vi "FUG_MagnetPS.destructor.vi"(0 "i ref in":refnum<vi>, 5 "error in (no error)":errorcluster) -> (19 "error out":errorcluster)   [LabVIEW 2014, in "FUG_MagnetPS.lvlib"]
doc: "This is the destructor of a class.\n\nLicense Agreement for this software:\n\nCopyright (C)\nGesellschaft für Schwerionenforschung, GSI\nPlanckstr. 1\n64291 Darmstadt\nGermany\n\nContact: D.Beck@gsi.de \n\nThis program is free software; you can redistribute it and/or modify it under the terms of the \nGNU General Public License as published by the Free Software Foundation; either version 2 of \nthe license, or (at your option) any later version.\n\nThis program is distributed in the hope that it will be useful, but WITHOUT ANY WARRANTY; \nwithout even the implied warranty of MERCHANTABILITY or FITNESS FOR A PARTICULAR PURPOSE. See the GNU General License for more details (http://www.gnu.org).\n\nGesellschaft für Schwerionenforschung, GSI\nPlanckstr. 1, 64291 Darmstadt, Germany\nFor all questions and ideas contact: M.Richter@gsi.de, H.Brand@gsi.de or D.Beck@gsi.de.\nLast update: 16-JUN-2004"
uses:
  FUG_MagnetPS.lvlib
  CS_PowerSupply/DIMPowerSupply/DIMPowerSupply.lvlib
  CSlibraries-extern/DimLVEvent/LVDimInterface/LVDimInterface.lvlib
  CS_PowerSupply/FUG_PowerSupply/FUG_PowerSupply.lvlib
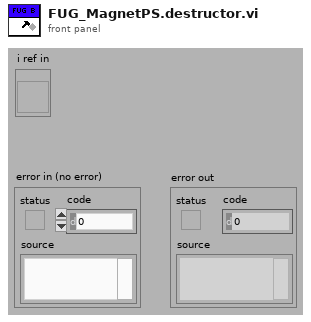
[diagram p1: front panel]
types:
  T1 = typedef "FUG_MagnetPS.lvlib/FUG_MagnetPS.i attribute.ctl" = cluster{"Gaussmeter":string, "SetField":dbl, "MagneticField queue":refnum<queue>, "Field Callback ID":i32, "nomCurrent":dbl, "Proportional":dbl, "Regulation?":bool, "actFieldID":i32, "nomFieldID":i32, "nomAutoCurrentID":i32, "regCurrentID":i32}
  T2 = enum16{"SetAttribute", "GetAttribute", "CreateAttribute", "DestroyAttribute", "DestroyAllAtributes"}
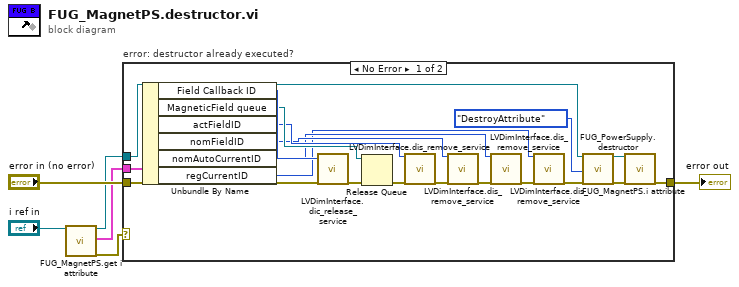
[diagram p0: block diagram]
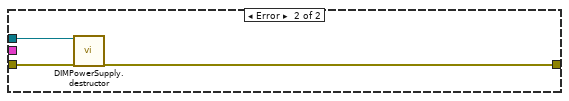
[diagram p2: hidden frame]
diagram:
  n1 = call "FUG_MagnetPS.get i attribute.vi"("i ref in"="i ref in") -> ("i ref out"=w2:refnum<vi>, "i attribute"=w1:T1, "error out"=w3:errorcluster)  [unwired: 16 in]
  n2 = case "error: destructor already executed?" shown="No Error" w3 {
    tunnel: [w22 w26] -> w6
    tunnel: "error in (no error)" -> [w19 w27]
    tunnel: w2 -> [w21 w28]
    tunnel: w1 -> [w20 _]
    frame No Error {
      n3 = Unbundle By Name(w20) -> ("Field Callback ID"=w18:i32, "MagneticField queue"=w16:refnum<queue>, "actFieldID"=w14:i32, "nomFieldID"=w11:i32, "nomAutoCurrentID"=w10:i32, "regCurrentID"=w7:i32)
      n4 = call "LVDimInterface.dic_release_service.vi"("callBackID"=w18, "error in (no error)"=w19) -> ("error out"=w17:errorcluster)  [unwired: 17 in]
      n5 = Release Queue(queue=w16, error in (no error)=w17) -> (error out=w15:errorcluster)  [unwired: 1 in, 2 out]
      n6 = call "LVDimInterface.dis_remove_service.vi"("my_serviceID"=w14, "error in (no error)"=w15) -> ("error out"=w13:errorcluster)  [unwired: 17 in]
      n7 = call "LVDimInterface.dis_remove_service.vi"("my_serviceID"=w11, "error in (no error)"=w13) -> ("error out"=w12:errorcluster)  [unwired: 17 in]
      n8 = call "LVDimInterface.dis_remove_service.vi"("my_serviceID"=w10, "error in (no error)"=w12) -> ("error out"=w9:errorcluster)  [unwired: 17 in]
      n9 = call "LVDimInterface.dis_remove_service.vi"("my_serviceID"=w7, "error in (no error)"=w9) -> ("error out"=w8:errorcluster)  [unwired: 17 in]
      n10 = call "FUG_MagnetPS.i attribute.vi"("VI Refnum"=w21, "Action"=T2."DestroyAttribute", "error in (no error)"=w8) -> ("VI Refnum out"=w24:refnum<vi>, "error out"=w23:errorcluster)  [unwired: 14 in, 1 out]
      n11 = call "FUG_PowerSupply.destructor.vi"("i ref in"=w24, "error in(no error)"=w23) -> ("error out"=w22:errorcluster)  [unwired: 17 in]
    }
    frame Error {
      n12 = call "DIMPowerSupply.destructor.vi"("i ref in"=w28, "error in (no error)"=w27) -> ("error out"=w26:errorcluster)  [unwired: 17 in]
    }
  }
  "error out" <- w6
